vi "IT8800-Default Instrument Setup.vi"(8 "error in":errorcluster, 11 "IT8800 Setting In In":T1={"VISA Resource Name"="", "Baud Rate"=19200, "Stop Bits"=20, "Wait For Read(ms)"=0, "Interface Type"=enum."VXI", "Limits"=[]} {"Stop Bits" items=["1.0"=10, "2.0"=20]; "Baud Rate" items=["2400"=2400, "4800"=4800, "9600"=9600, "19200"=19200]}) -> (0 "error out":errorcluster, 3 "IT8800 Setting In Out":T1={"VISA Resource Name"="", "Baud Rate"=19200, "Stop Bits"=20, "Wait For Read(ms)"=0, "Interface Type"=enum."VXI", "Limits"=[]} {"Stop Bits" items=["1.0"=10, "2.0"=20]; "Baud Rate" items=["2400"=2400, "4800"=4800, "9600"=9600, "19200"=19200]})   [LabVIEW 2018]
uses:
  Data Def/IT8800-Setting.ctl
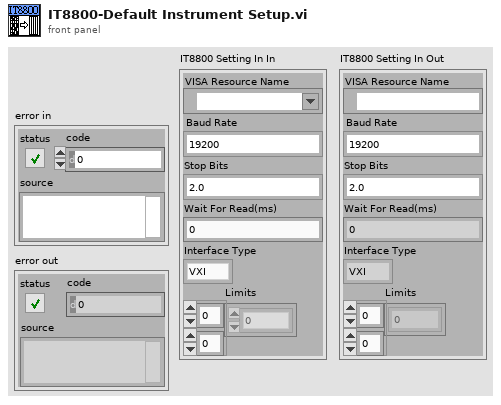
[diagram p1: front panel]
types:
  T1 = typedef "IT8800-Setting.ctl" = cluster{"VISA Resource Name":refnum<visa-resource-name>, "Baud Rate":u32, "Stop Bits":u16, "Wait For Read(ms)":u32, "Interface Type":enum16{"Unknow", "GPIB", "VXI", "GPIB-VXI", "Serial", "PXI", "TCPIP", "USB", "FireWire"}, "Limits":dbl[][]}
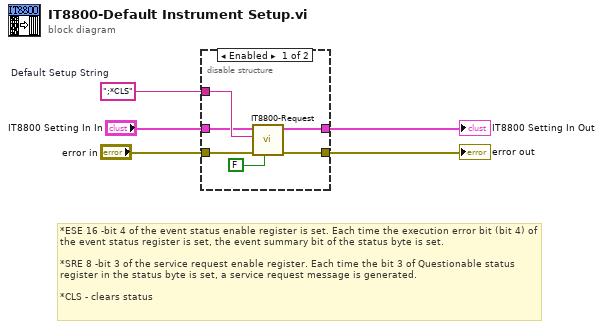
[diagram p0: block diagram]
diagram:
  w5 = ";*CLS"  # Default Setup String
  # "*ESE 16 -bit 4 of the event status enable register is set. Each time the execution error bit (bit 4) of the event status register is set, the event summary bit of the status byte is set.\n\n*SRE 8 -bit 3 of the service request enable register. Each time the bit 3 of Questionable status register in the status byte is set, a service request message is generated. \n\n*CLS - clears status"
  n1 = disable-structure shown="Enabled" {
    disable-tunnel: w5 -> [w11 _]
    disable-tunnel: "error in" -> [w10 w12]
    disable-tunnel: [w9 w12] -> w3
    disable-tunnel: "IT8800 Setting In In" -> [w8 w13]
    disable-tunnel: [w7 w13] -> w1
    frame Enabled {
      n2 = call "IT8800-Request.vi"("Response?"=FALSE, "error in"=w10, "Command"=w11, "IT8800 Setting In In"=w8) -> ("error out"=w9:errorcluster, "IT8800 Setting In Out"=w7:T1)  [unwired: 5 in, 1 out]
    }
    frame Disabled {
    }
  }
  "error out" <- w3
  "IT8800 Setting In Out" <- w1
